vi "WaveformGraph.vi"() -> ()   [LabVIEW 2013]
uses:
  <vilib>/Utility/miscctls.llb/LVPointDoubleTypeDef.ctl
panel:
  out "Waveform Graph":dbl[](graph)
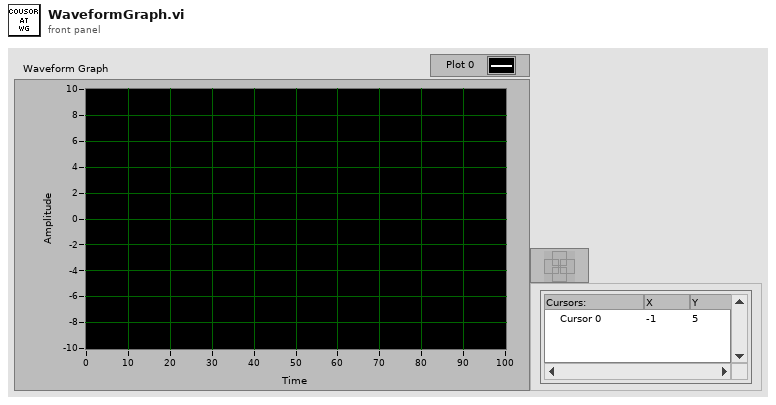
[diagram p1: front panel]
types:
  T1 = typedef "LVPointDoubleTypeDef.ctl" = cluster{"X":dbl, "Y":dbl}
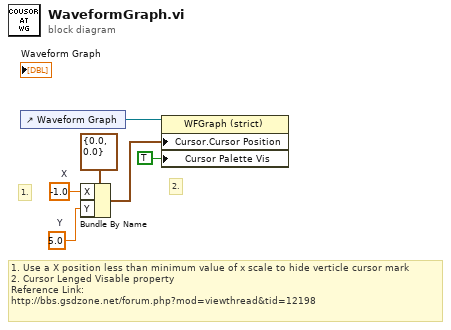
[diagram p0: block diagram]
diagram:
  w2 = 5.0  # Y
  w3 = -1.0  # X
  # "1. Use a X position less than minimum value of x scale to hide verticle cursor mark\n2. Cursor Lenged Visable property\nReference Link:\nhttp://bbs.gsdzone.net/forum.php?mod=viewthread&tid=12198"
  # "2."
  # "1."
  n1 = control-ref of="Waveform Graph"() -> (w6:refnum<vi>)
  n2 = Bundle By Name(cluster=T1 {"X"=0.0, "Y"=0.0} ("Cursor.Cursor Position"), "X"=w3, "Y"=w2) -> (w4:T1)
  n3 = property class="WFGraph (strict)"(reference=w6, "Cursor.Cursor Position"=w4, "Cursor Palette Vis"=TRUE ("Cursor Legend Visible")) -> ()  [unwired: 1 in, 2 out]
